vi "Arttu_v09_97.vi"() -> ()   [LabVIEW 2016]
uses:
  x64/Debug/BERTTA.dll
panel:
  out "element":bool
  out "Started:":string
  in  "SHUTDOWN":bool
  in  "MASTER CONTROL":bool
  in  "Tab Control":T1(tab)
  out "Output File":path caption="selected path"
  in  "Browse folder":path=path "" caption="start path"
  in  "Read Seq":bool
  in  "Save Seq":bool
  in  "Configuration file":path=path "C:/Users/shresplab/Desktop/ArttuConfiguration.lvm" caption="Filename"
  in  "OK Button 2":bool
  out "Boolean":bool
  in  "User (initials)":string
  in  "Project name":string
  in  "Description":string
  out "PUMP1":bool
  out "Target amount":dbl
  out "Scale weight":dbl
  out "Amount now":dbl
  out "Flow rate":dbl
  out "Time to target":dbl format="%<%H:%M:%S>t"
  out "Current step":dbl
  out "Target":dbl
  out "Amount now":dbl
  out "Amount now":dbl
  out "Target":dbl
  out "Current step":dbl
  out "Time to target":dbl format="%<%H:%M:%S>t"
  out "Flow rate":dbl
  out "Amount now":dbl
  out "Scale weight":dbl
  out "Target amount":dbl
  out "PUMP2":bool
  out "Sensor OK 6":bool
  out "Sensor OK 5":bool
  out "Sensor OK 4":bool
  out "Sensor OK 3":bool
  in  "OK Button":bool
  in  "Add comment":string
  out "PUMP3":bool
  out "Target amount":dbl
  out "Scale weight":dbl
  out "Amount now":dbl
  out "Flow rate":dbl
  out "Time to target":dbl format="%<%H:%M:%S>t"
  out "Current step":dbl
  out "Target":dbl
  out "Amount now":dbl
  out "Tr":dbl
  out "Tj in":dbl
  out "Tj out":dbl
  out "T set":dbl
  out "Current step":i32
  out "RPM":dbl
  out "Torque 2":dbl
  out "Waveform Chart 5":dynamicdata(graph)
  out "Waveform Chart 6":dynamicdata(graph)
  out "Waveform Chart 7":dynamicdata(graph)
  in  "Tab Control 2":T2(tab)
  out "Waveform Chart 3":dynamicdata(graph)
  out "Waveform Chart 8":dynamicdata(graph)
  out "Waveform Chart 11":dynamicdata(graph)
  out "Waveform Chart 13":dynamicdata(graph)
  out "Waveform Chart 9":dynamicdata(graph)
  out "Table":string[][](table)=[["14.8.2017 18.06.59", "0,000000", "417,670000", "-0,150000", "1,000000", "22,220000", "23,366837", "23,574959", "23,985852", "23,690000", "240,000000", "4,000000", "0,000000", "397,000000", "-397,000000", "1,000000"], ["14.8.2017 18.07.06", "0,000000", "417,640000", "-0,120000", "1,000000", "22,220000", "23,763115", "23,906257", "23,985694", "23,680000", "240,000000", "4,000000", "0,000000", "397,000000", "-397,000000", "1,000000"], ["14.8.2017 18.07.13", "0,000000", "417,640000", "-0,120000", "1,000000", "22,220000", "23,965922", "24,013440", "23,984906", "23,670000", "240,000000", "4,100000", "3,000000", "397,000000", "-397,000000", "1,000000"], ["14.8.2017 18.07.21", "0,000000", "417,640000", "-0,120000", "1,000000", "22,220000", "23,943860", "23,900110", "23,987113", "23,670000", "240,000000", "4,000000", "0,000000", "397,000000", "-397,000000", "1,000000"], ["14.8.2017 18.07.28", "0,000000", "417,640000", "-0,120000", "1,000000", "22,220000", "23,736328", "23,600018", "23,989004", "23,660000", "240,000000", "4,000000", "0,000000", "397,000000", "-397,000000", "1,000000"], ["14.8.2017 18.07.36", "0,000000", "417,640000", "-0,120000", "1,000000", "22,220000", "23,480910", "23,324538", "23,991053", "23,660000", "240,000000", "4,000000", "0,000000", "397,000000", "-397,000000", "1,000000"], ["14.8.2017 18.07.43", "0,000000", "417,640000", "-0,120000", "2,000000", "22,220000", "23,195579", "23,008270", "23,999093", "23,650000", "240,000000", "4,000000", "0,000000", "397,000000", "-397,000000", "1,000000"], ["14.8.2017 18.07.51", "0,000000", "417,650000", "-417,650000", "1,000000", "22,220000", "22,862541", "22,649021", "24,003979", "23,650000", "240,000000", "4,000000", "0,000000", "397,000000", "-397,000000", "2,000000"], ["14.8.2017 18.07.58", "0,000000", "417,640000", "0,010000", "1,000000", "22,220000", "22,541353", "22,354878", "24,005398", "23,650000", "240,000000", "4,000000", "0,000000", "397,000000", "-397,000000", "1,000000"], ["14.8.2017 18.08.06", "0,000000", "417,640000", "0,010000", "1,000000", "22,220000", "22,347931", "22,253738", "24,007605", "23,640000", "240,000000", "4,100000", "0,000000", "397,000000", "-397,000000", "1,000000"], ["14.8.2017 18.08.13", "0,000000", "417,640000", "0,010000", "1,000000", "22,220000", "22,329030", "22,302102", "24,006028", "23,640000", "240,000000", "4,000000", "0,000000", "395,820000", "-395,820000", "1,000000"], ["14.8.2017 18.08.20", "0,000000", "417,640000", "0,010000", "1,000000", "22,220000", "22,466849", "22,511320", "24,002403", "23,630000", "240,000000", "4,000000", "0,000000", "395,830000", "-0,010000", "1,000000"], ["14.8.2017 18.08.28", "0,000000", "417,640000", "0,010000", "1,000000", "22,220000", "22,707062", "22,835101", "24,000984", "23,620000", "240,000000", "4,000000", "0,000000", "395,830000", "-0,010000", "1,000000"], ["14.8.2017 18.08.35", "0,000000", "417,640000", "0,010000", "1,000000", "22,220000", "23,054104", "23,232979", "24,001299", "23,600000", "240,000000", "4,000000", "0,000000", "395,830000", "-0,010000", "1,000000"], ["14.8.2017 18.08.43", "0,000000", "417,640000", "0,010000", "1,000000", "22,220000", "23,412371", "23,522793", "24,002560", "23,590000", "240,000000", "4,000000", "0,000000", "395,820000", "0,000000", "1,000000"], ["14.8.2017 18.08.51", "0,000000", "417,640000", "0,010000", "1,000000", "22,220000", "23,596247", "23,656125", "24,003821", "23,580000", "240,000000", "4,000000", "0,000000", "395,820000", "0,000000", "1,000000"]]
  out "Boolean 4":bool
  out "Boolean 3":bool
  out "Boolean 2":bool
  in  "Reset 6":bool
  in  "Manual/Ramp":bool=TRUE
  in  "Array":dbl[][](array[numeric])=[[20.0, 0.0], [20.0, 0.0], [20.0, 0.0]]
  in  "?":bool
  in  "Time":dbl format="Time to target (min):                %#_g"
  out "Current temp":dbl format="Current temperature (S1):   %#_6g"
  in  "OK Button 3":bool
  in  "T ext / T ext 2":enum32{"Sensor 1", "Sensor 2"}(radio)
  out "Sensor OK":bool
  in  "T fail":dbl=20.0 format="Failsafe temperature:              %#_g"
  in  "Setpoint":dbl=20.0 format="Temperature target:                %#_6g"
  in  "Manual select":T3(radio)
  out "Waveform Chart":dynamicdata(graph)
  out "T external 2":dbl format="Current temperature (S2):    %#_g"
  in  "UPDATE TEMP":bool
  out "Led11 5":bool
  out "RPM":dbl format="%_4f"
  out "Led10 3":bool
  out "Led9 3":bool
  out "Led8 3":bool
  out "Led7 3":bool
  out "Led6 3":bool
  out "Led5 3":bool
  out "Led4 3":bool
  out "Led3 3":bool
  out "Led2 3":bool
  out "Led1 3":bool
  in  "PumpSeq 4":dbl[][](array[numeric])=[[0.0, 0.0, 0.0, 0.0, 0.0, 0.0, 0.0, 0.0, 0.0, 0.0], [0.0, 0.0, 0.0, 0.0, 0.0, 0.0, 0.0, 0.0, 0.0, 0.0], [0.0, 0.0, 0.0, 0.0, 0.0, 0.0, 0.0, 0.0, 0.0, 0.0], [0.0, 0.0, 0.0, 0.0, 0.0, 0.0, 0.0, 0.0, 0.0, 0.0], [0.0, 0.0, 0.0, 0.0, 0.0, 0.0, 0.0, 0.0, 0.0, 0.0], [0.0, 0.0, 0.0, 0.0, 0.0, 0.0, 0.0, 0.0, 0.0, 0.0], [0.0, 0.0, 0.0, 0.0, 0.0, 0.0, 0.0, 0.0, 0.0, 0.0], [0.0, 0.0, 0.0, 0.0, 0.0, 0.0, 0.0, 0.0, 0.0, 0.0], [0.0, 0.0, 0.0, 0.0, 0.0, 0.0, 0.0, 0.0, 0.0, 0.0], [0.0, 0.0, 0.0, 0.0, 0.0, 0.0, 0.0, 0.0, 0.0, 0.0]]
  in  "?":bool
  out "Flow rate (g/min)":dbl
  out "Scale reading":dbl
  out "Step amount now":dbl
  in  "Grams / min":dbl
  out "Waveform Chart 14":dynamicdata(graph)
  in  "?":bool
  out "Total amount now":dbl
  out "Led11 4":bool
  in  "Reset 5":bool
  out "Elapsed / step":i32
  out "Time to target":dbl format="%<%H:%M:%S>t"
  in  "OK Button 4":bool
  out "Led11":bool
  out "RPM":dbl format="%_4f"
  out "Led10":bool
  out "Led9":bool
  out "Led8":bool
  out "Led7":bool
  out "Led6":bool
  out "Led5":bool
  out "Led4":bool
  out "Led3":bool
  out "Led2":bool
  out "Led1":bool
  in  "PumpSeq 2":dbl[][](array[numeric])=[[0.0, 0.0, 0.0, 0.0, 0.0, 0.0, 0.0, 0.0, 0.0, 0.0], [0.0, 0.0, 0.0, 0.0, 0.0, 0.0, 0.0, 0.0, 0.0, 0.0], [0.0, 0.0, 0.0, 0.0, 0.0, 0.0, 0.0, 0.0, 0.0, 0.0], [0.0, 0.0, 0.0, 0.0, 0.0, 0.0, 0.0, 0.0, 0.0, 0.0], [0.0, 0.0, 0.0, 0.0, 0.0, 0.0, 0.0, 0.0, 0.0, 0.0], [0.0, 0.0, 0.0, 0.0, 0.0, 0.0, 0.0, 0.0, 0.0, 0.0], [0.0, 0.0, 0.0, 0.0, 0.0, 0.0, 0.0, 0.0, 0.0, 0.0], [0.0, 0.0, 0.0, 0.0, 0.0, 0.0, 0.0, 0.0, 0.0, 0.0], [0.0, 0.0, 0.0, 0.0, 0.0, 0.0, 0.0, 0.0, 0.0, 0.0], [0.0, 0.0, 0.0, 0.0, 0.0, 0.0, 0.0, 0.0, 0.0, 0.0]]
  in  "?":bool
  out "Flow rate (g/min)":dbl
  out "Scale reading":dbl
  out "Step amount now":dbl
  in  "Grams / min":dbl
  out "Waveform Chart 10":dynamicdata(graph)
  in  "?":bool
  out "Total amount now":dbl
  out "Led11":bool
  in  "Reset 3":bool
  out "Elapsed / step":i32
  out "Time to target":dbl format="%<%H:%M:%S>t"
  in  "OK Button 5":bool
  out "Led11 3":bool
  out "RPM":dbl format="%_4f"
  out "Led10 2":bool
  out "Led9 2":bool
  out "Led8 2":bool
  out "Led7 2":bool
  out "Led6 2":bool
  out "Led5 2":bool
  out "Led4 2":bool
  out "Led3 2":bool
  out "Led2 2":bool
  out "Led1 2":bool
  in  "PumpSeq 3":dbl[][](array[numeric])=[[0.0, 0.0, 0.0, 0.0, 0.0, 0.0, 0.0, 0.0, 0.0, 0.0], [0.0, 0.0, 0.0, 0.0, 0.0, 0.0, 0.0, 0.0, 0.0, 0.0], [0.0, 0.0, 0.0, 0.0, 0.0, 0.0, 0.0, 0.0, 0.0, 0.0], [0.0, 0.0, 0.0, 0.0, 0.0, 0.0, 0.0, 0.0, 0.0, 0.0], [0.0, 0.0, 0.0, 0.0, 0.0, 0.0, 0.0, 0.0, 0.0, 0.0], [0.0, 0.0, 0.0, 0.0, 0.0, 0.0, 0.0, 0.0, 0.0, 0.0], [0.0, 0.0, 0.0, 0.0, 0.0, 0.0, 0.0, 0.0, 0.0, 0.0], [0.0, 0.0, 0.0, 0.0, 0.0, 0.0, 0.0, 0.0, 0.0, 0.0], [0.0, 0.0, 0.0, 0.0, 0.0, 0.0, 0.0, 0.0, 0.0, 0.0], [0.0, 0.0, 0.0, 0.0, 0.0, 0.0, 0.0, 0.0, 0.0, 0.0]]
  in  "?":bool
  out "Flow rate (g/min)":dbl
  out "Scale reading":dbl
  out "Step amount now":dbl
  in  "Grams / min":dbl
  out "Waveform Chart 12":dynamicdata(graph)
  in  "?":bool
  out "Total amount now":dbl
  out "Led11 2":bool
  in  "Reset 4":bool
  out "Elapsed / step":i32
  out "Time to target":dbl format="%<%H:%M:%S>t"
  in  "OK Button 6":bool
  in  "?":bool
  in  "Scale port":dbl=3.0
  out "Waveform Chart 15":dynamicdata(graph)
  in  "?":bool
  in  "OK Button 8":bool
  in  "Remote / Manual":bool
  in  "Set RPM":i32
  out "RPM":dbl
  out "Torque":dbl
  out "Waveform Chart 4":dynamicdata(graph)
  in  "OK Button 7":bool
  out "PortDev out":dbl[](array[numeric])
  in  "Save PortDev":bool
  out "PortDev in":dbl[](array[numeric])
  in  "dev1":i32
  in  "dev2":i32
  in  "dev3":i32
  in  "dev4":i32
  in  "dev5":i32
  in  "dev6":i32
  in  "dev8":i32
  in  "port1":i32
  in  "port2":i32
  in  "port3":i32
  in  "port4":i32
  in  "port5":i32
  in  "port6":i32
  in  "port7":i32
  in  "port8":i32
  in  "dev7":i32
  in  "Treshold (T/C)":dbl=0.5
  out "DAQ 9217 (PT100)":errorcluster
  out "Config File":dbl[][](array[numeric])
  in  "Temp Control":tag="cDAQ9188XT-1C3BEFEMod1"
  in  "PAM Control":tag="cDAQ9188XT-1C3BEFEMod7"
  # "Temperature sensor:"
  # "Manual control:"
  # "PUMP & SCALE 1"
  # "STEP"
  # "TOTAL"
  # "PUMP & SCALE 2"
  # "STEP"
  # "TOTAL"
  # "PUMP & SCALE 3"
  # "STEP"
  # "TOTAL"
  # "Temperature control parameter"
  # "Secondary temperature sensor"
  # "Temp target"
  # "Time target"
  # "Grams    /   min"
  # "End of sequence"
  # "Manual control"
  # "Grams    /   min"
  # "End of sequence"
  # "Manual control"
  # "Grams    /   min"
  # "End of sequence"
  # "Manual control"
  # "PAM control"
  # "dev1 and dev2 always to port1 and 2\nport1 = port2 = Lauda\n\ndev3 and dev4 always to port3 and port4\nport3 = port4 = Heidolph"
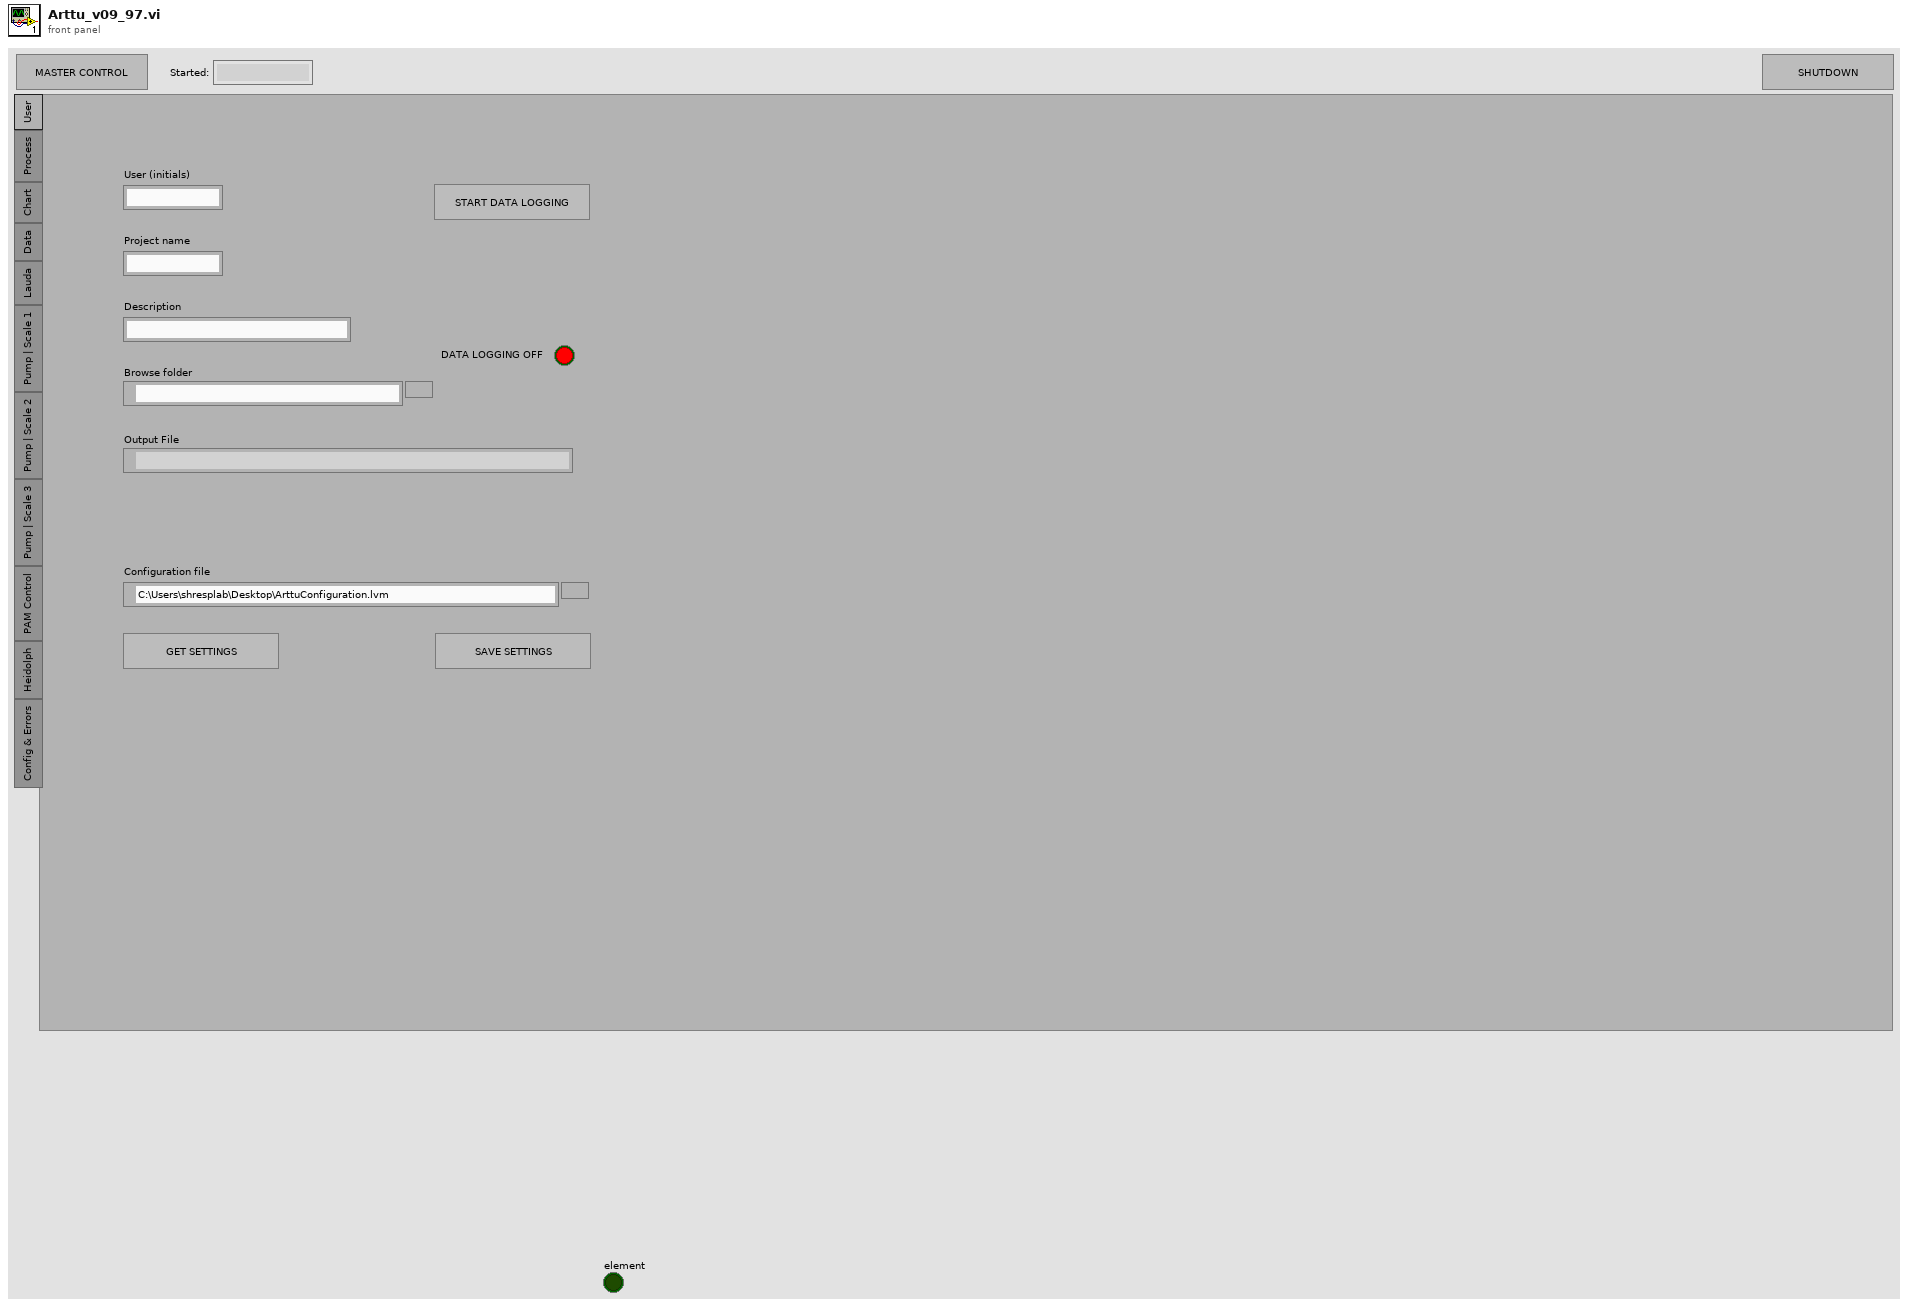
[diagram p1: front panel]
types:
  T1 = enum32{"User", "Process", "Chart", "Data", "Lauda", "Pump | Scale 1", "Pump | Scale 2", "Pump | Scale 3", "PAM Control", "Heidolph", "Config & Errors"}
  T2 = enum32{"Temperatures", "Scale / Pump 1", "Scale / Pump 2", "Scale / Pump 3", "RPM / torque"}
  T3 = enum32{"Reactor temperature", "Jacket temperature"}
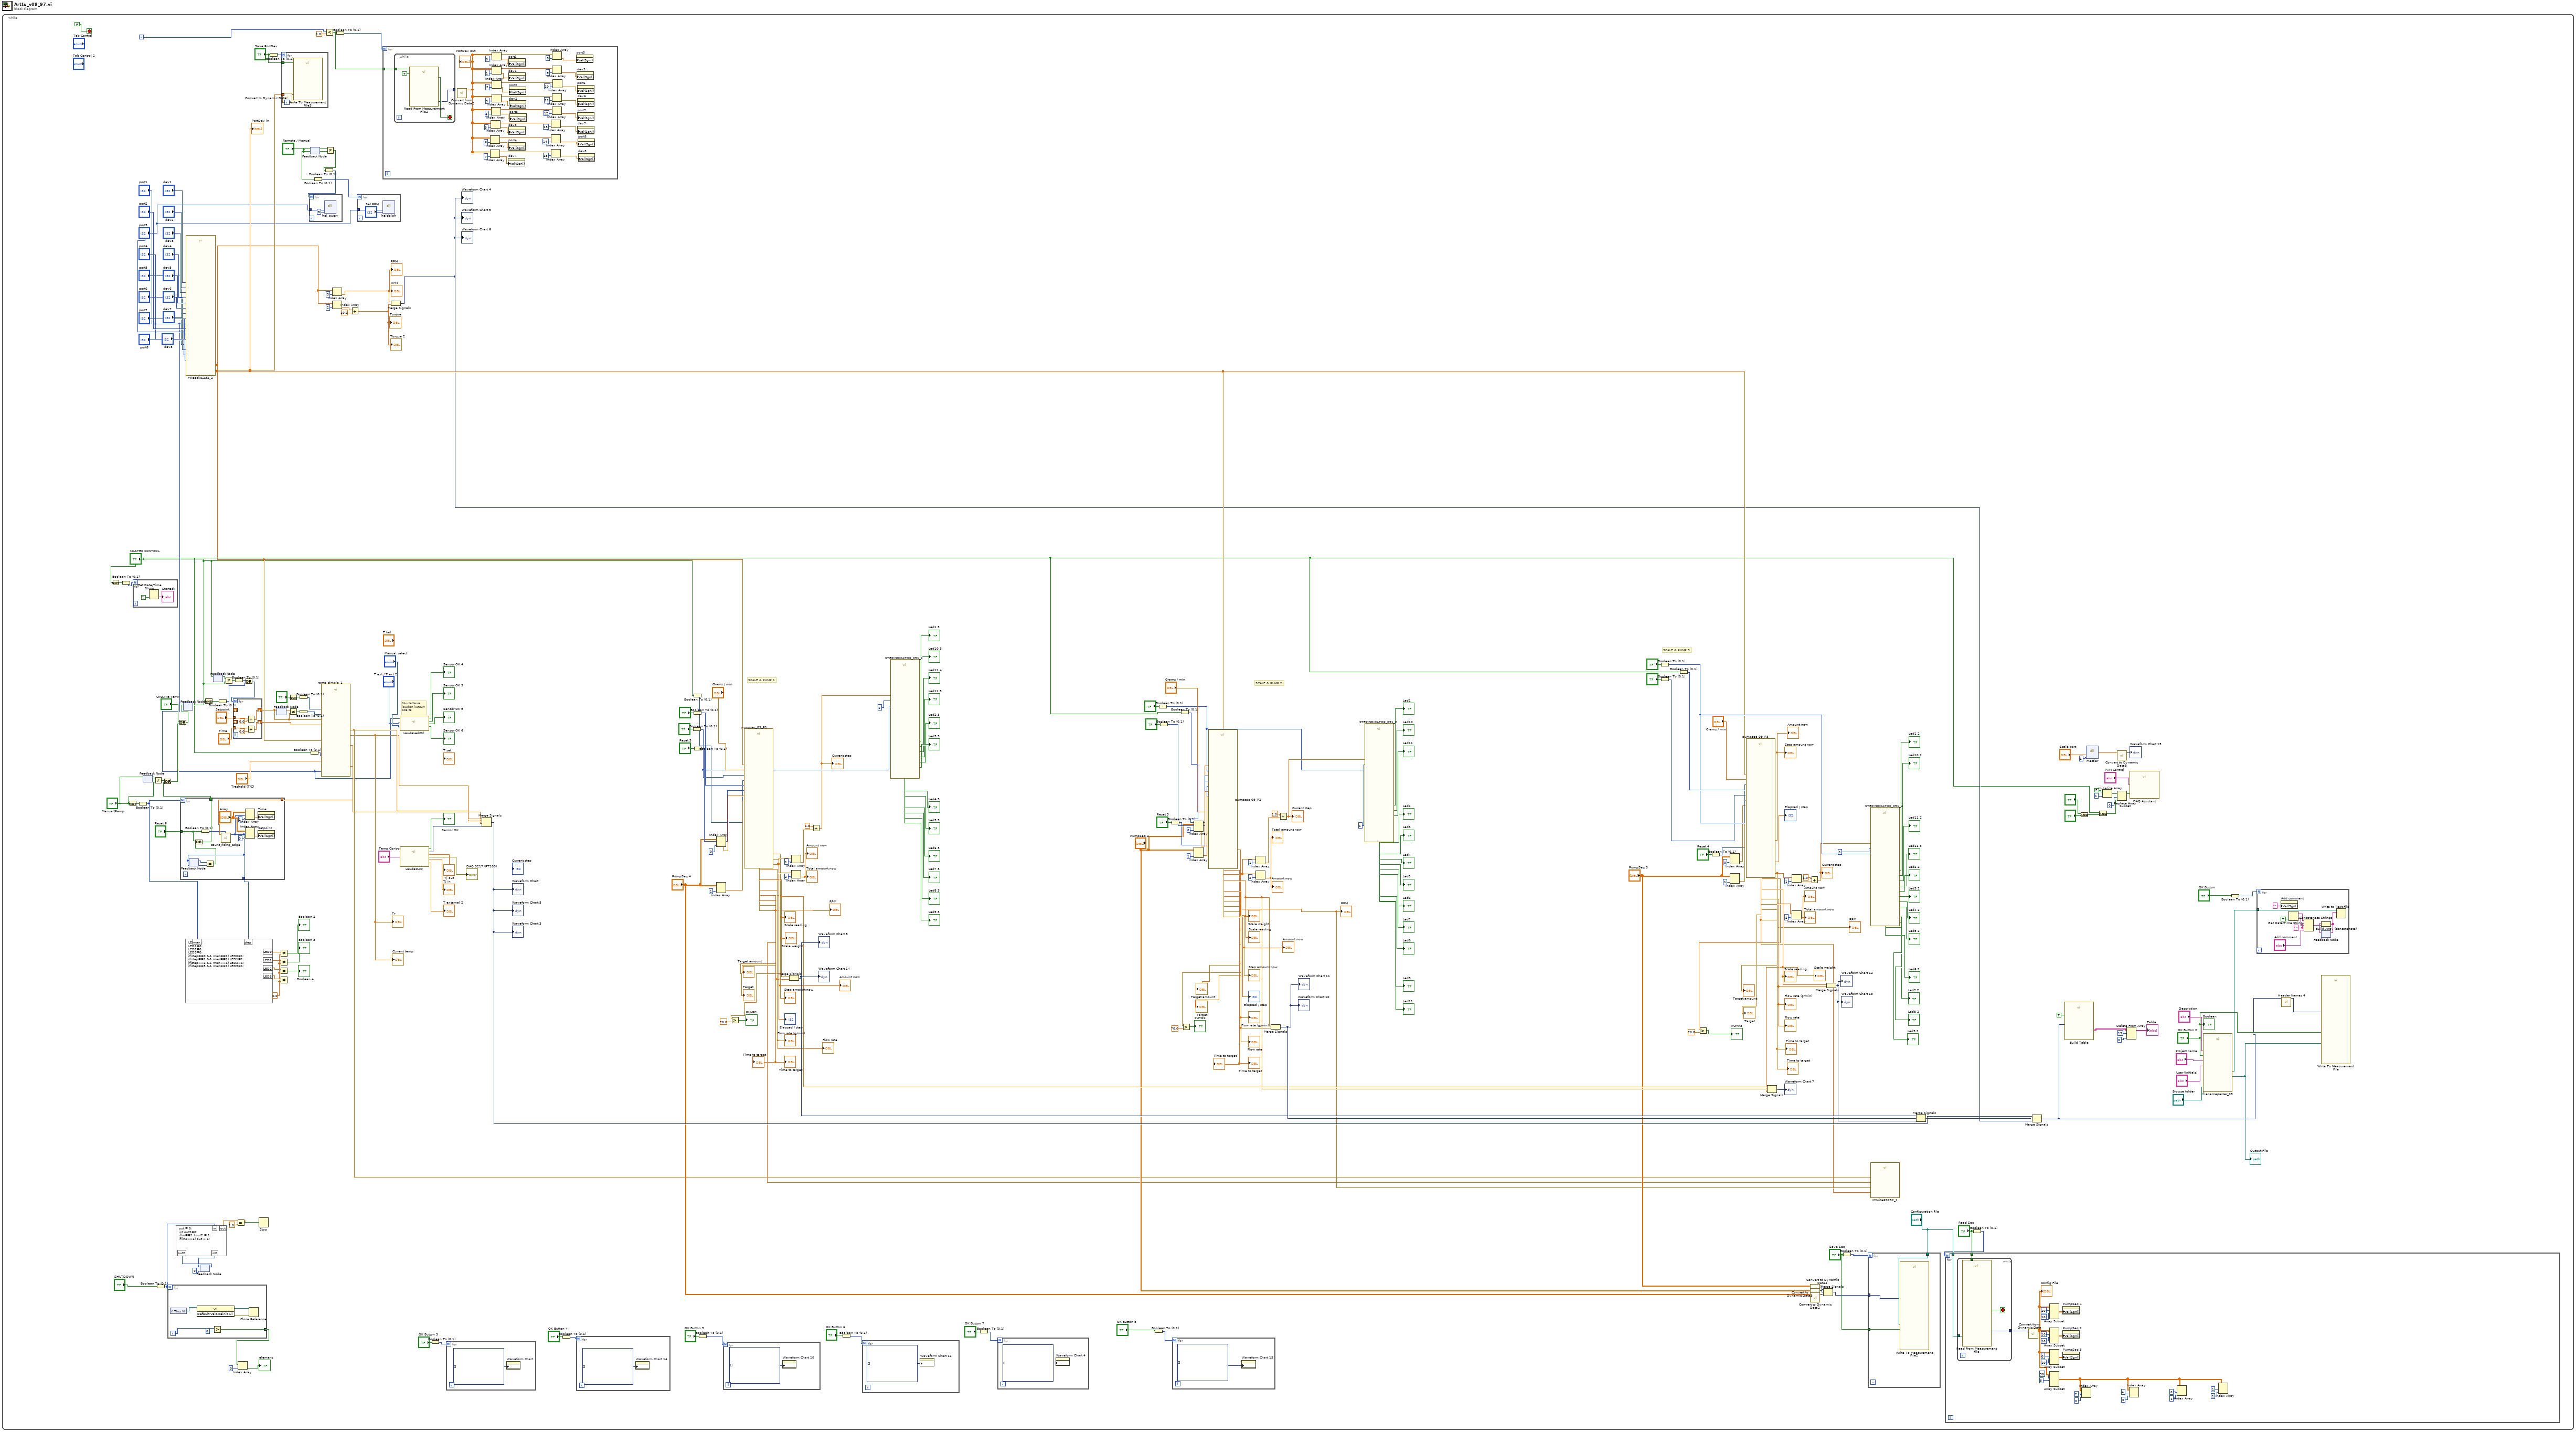
[diagram p0: block diagram]
diagram:
  n1 = while {
    i -> [w61]
    stop <- FALSE stop-if-true
    w47 = 0.0 ("y")
    # "Muutettava\nlaudan kutsun \nosalta"
    # "SCALE & PUMP 1"
    # "SCALE & PUMP 3"
    # "SCALE & PUMP 2"
    n2 = Not(x="MASTER CONTROL") -> (.not. x?=w290:bool)
    n3 = Boolean To (0,1)(Boolean=w290) -> (0, 1=w291:i16)
    n4 = Not(x="Manual/Ramp") -> (.not. x?=w54:bool)
    n5 = for {
      N: w291 -> [_]
      n6 = Get Date/Time String(want seconds? (F)=TRUE) -> (time string=→"Started:":string)  [unwired: 2 in, 1 out]
    }
    n7 = Boolean To (0,1)(Boolean=w54) -> (0, 1=w36:i16)
    n8 = feedback #1() -> (w42:bool)  [unwired: 1 in]
    n9 = feedback-in #1("Manual/Ramp") -> ()
    n10 = Not Equal?(x=w42, y="Manual/Ramp") -> (x != y?=w39:bool)
    n11 = Boolean To (0,1)(Boolean="SHUTDOWN") -> (0, 1=w275:i16)
    n12 = for {
      N: w275 -> [_]
      tunnel: [w407] -> w289 mode=indexing
      i -> [w409]
      n13 = control-ref of="This VI"() -> (w412:refnum<vi>)
      n14 = invoke class="VI" method="Default Vals.Reinit All"(reference=w412) -> (reference out=w410:refnum<vi>, error out=w411:errorcluster)  [unwired: 2 in, 1 out]
      n15 = Greater?(x=w409, y=0) -> (0:w407:bool)
      n16 = Close Reference(reference=w410, error in (no error)=w411) -> ()  [unwired: 1 out]
    }
    n17 = feedback #2() -> (w34:bool)  [unwired: 1 in]
    n18 = call "MReadRS232_2.vi"("port1"="port1", "dev1"="dev1", "port2"="port2", "dev2"="dev2", "port3"="port3", "dev7"="dev7", "dev8"="dev8", "port7"="port7", "port8"="port8", "dev5"="dev5", "port5"="port5", "dev4"="dev4", "dev6"="dev6", "port6"="port6", "port4"="port4", "dev3"="dev3") -> ("output array"=w65:dbl[], "params"=w26:dbl[])  [unwired: 2 in]
    "PortDev in" <- w65
    n19 = feedback #3(0) -> (w273:i32)
    n20 = formula code="out = 0;\nint out2=0;\nif(in==1 ) out2 = 1;\nif(in2==1) out = 1;"("in"=w275, "in2"=w273) -> ("out"=w277:dbl, "out2"=w274:i32)
    n21 = feedback-in #3(w274) -> ()
    n22 = And(x="MASTER CONTROL", y=w34) -> (x .and. y?=w92:bool)
    n23 = feedback #4() -> (w83:bool)  [unwired: 1 in]
    n24 = feedback-in #4("MASTER CONTROL") -> ()
    n25 = Boolean To (0,1)(Boolean=w92) -> (0, 1=w81:i16)
    n26 = Not Equal?(x=w83, y="MASTER CONTROL") -> (x != y?=w82:bool)
    n27 = Boolean To (0,1)(Boolean=w82) -> (0, 1=w80:i16)
    n28 = Equal?(x=w277, y=1.0) -> (x = y?=w276:bool)
    n29 = Index Array(array=w289, index=0) -> (element=→"element":bool)
    n30 = Or(x=w80, y=w81) -> (x .or. y?=w79:i16)
    n31 = for {
      N: w79 -> [_]
      tunnel: "Time" -> [w359]
      shift-right: [w358] -> w93
      shift-left: _ -> [_]
      tunnel: "Setpoint" -> [w356]
      shift-right: [w355] -> w90
      shift-left: _ -> [_]
      n32 = Add(x=w356, y=0.0) -> (x+y=w355:dbl)
      n33 = Add(x=w359, y=0.0) -> (x+y=w358:dbl)
    }
    n34 = Stop(stop? (T)=w276) -> ()
    n35 = Boolean To (0,1)(Boolean="Save PortDev") -> (0, 1=w64:i16)
    n36 = feedback-in #5(w90) -> ()
    n37 = feedback #5() -> (w91:dbl)  [unwired: 1 in]
    n38 = for {
      N: w64 -> [_]
      tunnel: w65 -> [w354]
      tunnel: "Save PortDev" -> [w352]
      n39 = call "Convert to Dynamic Data"("Array"=w354) -> ("Dynamic Data Type"=w353:dynamicdata)  [unwired: 3 in]
      n40 = call "Write To Measurement File3"("Signals"=w353, "Reset"=w352) -> ()  [unwired: 15 in, 3 out]
    }
    n41 = Not(x="?") -> (.not. x?=w86:bool)
    n42 = Not Equal?(x=w91, y=w90) -> (x != y?=w89:bool)
    n43 = Boolean To (0,1)(Boolean=w86) -> (0, 1=w88:i16)
    n44 = Boolean To (0,1)(Boolean=w89) -> (0, 1=w84:i16)
    n45 = Boolean To (0,1)(Boolean="MASTER CONTROL") -> (0, 1=w85:i16)
    n46 = feedback-in #6("Remote / Manual") -> ()
    n47 = feedback #6() -> (w31:bool)  [unwired: 1 in]
    n48 = Boolean To (0,1)(Boolean="Remote / Manual") -> (0, 1=w29:i16)
    n49 = call "ramp_simple_1.vi"("pause"=w88, "time_set"=w93, "array"=w26, "reset"=w84, "master"=w85, "T_sp"=w90, "treshold"="Treshold (T/C)", "port"="port1") -> ("Tin"=w96:dbl, "Tr"=w97:dbl, "target_reached"=w52:dbl, "T control"=w98:dbl)  [unwired: 3 in, 1 out]
    "Tr" <- w97
    "Current temp" <- w97
    n50 = for {
      N: w36 -> [_]
      tunnel: w52 -> [w311]
      tunnel: [w301] -> w40
      tunnel: "Reset 6" -> [w303]
      tunnel: [w304] -> w43
      n51 = feedback #7() -> (w305:i32)  [unwired: 1 in]
      n52 = Boolean To (0,1)(Boolean=w303) -> (0, 1=w306:i16)
      n53 = call "count_rising_edge.vi"("reset"=w306, "target_reached"=w311) -> ("element 2"=w304:i32)  [unwired: 9 in]
      n54 = feedback-in #7(w304) -> ()
      n55 = Not Equal?(x=w305, y=w304) -> (x != y?=w302:bool)
      n56 = Or(x=w303, y=w302) -> (x .or. y?=w301:bool)
      n57 = Index Array(array="Array", index (row)=w304, index (col)=1 ("disabled index (col)")) -> (element=w307:dbl)
      n58 = Index Array(array="Array", index (row)=w304, index (col)=0 ("disabled index (col)")) -> (element=w308:dbl)
      n59 = property on="Time" class="DigNum (strict)"("Val(Sgnl)"=w307) -> ()  [unwired: 2 in, 2 out]
      n60 = property on="Setpoint" class="DigNum (strict)"("Val(Sgnl)"=w308) -> ()  [unwired: 2 in, 2 out]
    }
    n61 = Or(x=w39, y=w40) -> (x .or. y?=w38:bool)
    n62 = Or(x="UPDATE TEMP", y=w38) -> (x .or. y?=w35:bool)
    n63 = feedback-in #2(w35) -> ()
    n64 = formula code="LED0=0;\nLED1=0;\nLED2=0;\nLED3=0;\nif(step==0 && man==1) LED0=1;\nif(step==1 && man==1) LED1=1;\nif(step==2 && man==1) LED2=1;\nif(step==3 && man==1) LED3=1;"("step"=w43, "man"=w36) -> ("LED0"=w51:dbl, "LED1"=w50:dbl, "LED2"=w49:dbl, "LED3"=w48:dbl)
    n65 = Not Equal?(x=w51, y=w47) -> (x != y?=→"Boolean 2":bool)
    n66 = Not Equal?(x=w50, y=w47) -> (x != y?=→"Boolean 3":bool)
    n67 = Not Equal?(x=w49, y=w47) -> (x != y?=→"Boolean 4":bool)
    n68 = Not Equal?(x=w48, y=w47) -> ()  [unwired: 1 out]
    n69 = Less?(x=w61, y=1.0) -> (x < y?=w59:bool)
    n70 = Not Equal?(x=w31, y="Remote / Manual") -> (x != y?=w30:bool)
    n71 = Boolean To (0,1)(Boolean=w30) -> (0, 1=w32:i16)
    n72 = for {
      N: w32 -> [_]
      tunnel: "port3" -> [w299]
      n73 = dll-call lib="C:/Users/shresplab/OneDrive - Kemira Oyj/Documents/GitHub/Bertta/BERTTA/x64/Debug/BERTTA.dll" fn="hei_query"("port"=w299, "q"=5) -> ()  [unwired: 6 in, 2 out]
    }
    n74 = Index Array(array=w26, index=3) -> (element=w23:dbl)
    "RPM" <- w23
    "RPM" <- w23
    n75 = Index Array(array=w26, index=2) -> (element=w25:dbl)
    n76 = Boolean To (0,1)(Boolean=w59) -> (0, 1=w60:i16)
    n77 = Divide(x=w25, y=10.0) -> (x/y=w22:dbl)
    "Torque" <- w22
    "Torque 2" <- w22
    n78 = for {
      N: w29 -> [_]
      tunnel: "port3" -> [w297]
      n79 = dll-call lib="C:/Users/shresplab/OneDrive - Kemira Oyj/Documents/GitHub/Bertta/BERTTA/x64/Debug/BERTTA.dll" fn="heidolph"("port"=w297, "speed"="Set RPM") -> ()  [unwired: 6 in, 2 out]
    }
    n80 = for {
      N: w60 -> [_]
      tunnel: w59 -> [w347]
      n81 = while {
        tunnel: [w350] -> w346
        tunnel: w347 -> [w348]
        stop <- w351 stop-if-true
        n82 = call "Read From Measurement File2"("Enable"=TRUE, "Reset"=w348) -> ("Signals"=w350:dynamicdata, "EOF?"=w351:bool)  [unwired: 4 in, 4 out]
      }
      n83 = call "Convert from Dynamic Data2"("Dynamic Data Type"=w346) -> ("Array"=w329:dbl[])  [unwired: 3 in]
      "PortDev out" <- w329
      n84 = Index Array(array=w329, index=6) -> (element=w322:dbl)
      n85 = Index Array(array=w329, index=7) -> (element=w321:dbl)
      n86 = Index Array(array=w329, index=5) -> (element=w323:dbl)
      n87 = Index Array(array=w329, index=4) -> (element=w324:dbl)
      n88 = Index Array(array=w329, index=0) -> (element=w328:dbl)
      n89 = Index Array(array=w329, index=1) -> (element=w327:dbl)
      n90 = Index Array(array=w329, index=3) -> (element=w325:dbl)
      n91 = Index Array(array=w329, index=2) -> (element=w326:dbl)
      n92 = property on="dev4" class="DigNum (strict)"("Val(Sgnl)"=w321) -> ()  [unwired: 2 in, 2 out]
      n93 = property on="dev3" class="DigNum (strict)"("Val(Sgnl)"=w323) -> ()  [unwired: 2 in, 2 out]
      n94 = property on="port4" class="DigNum (strict)"("Val(Sgnl)"=w322) -> ()  [unwired: 2 in, 2 out]
      n95 = property on="port1" class="DigNum (strict)"("Val(Sgnl)"=w328) -> ()  [unwired: 2 in, 2 out]
      n96 = property on="dev1" class="DigNum (strict)"("Val(Sgnl)"=w327) -> ()  [unwired: 2 in, 2 out]
      n97 = property on="port2" class="DigNum (strict)"("Val(Sgnl)"=w326) -> ()  [unwired: 2 in, 2 out]
      n98 = property on="dev2" class="DigNum (strict)"("Val(Sgnl)"=w325) -> ()  [unwired: 2 in, 2 out]
      n99 = property on="port3" class="DigNum (strict)"("Val(Sgnl)"=w324) -> ()  [unwired: 2 in, 2 out]
      n100 = Index Array(array=w329, index=14) -> (element=w314:dbl)
      n101 = Index Array(array=w329, index=15) -> (element=w313:dbl)
      n102 = Index Array(array=w329, index=13) -> (element=w315:dbl)
      n103 = Index Array(array=w329, index=12) -> (element=w316:dbl)
      n104 = Index Array(array=w329, index=8) -> (element=w320:dbl)
      n105 = Index Array(array=w329, index=9) -> (element=w319:dbl)
      n106 = Index Array(array=w329, index=11) -> (element=w317:dbl)
      n107 = Index Array(array=w329, index=10) -> (element=w318:dbl)
      n108 = property on="port5" class="DigNum (strict)"("Val(Sgnl)"=w320) -> ()  [unwired: 2 in, 2 out]
      n109 = property on="dev5" class="DigNum (strict)"("Val(Sgnl)"=w319) -> ()  [unwired: 2 in, 2 out]
      n110 = property on="port6" class="DigNum (strict)"("Val(Sgnl)"=w318) -> ()  [unwired: 2 in, 2 out]
      n111 = property on="dev6" class="DigNum (strict)"("Val(Sgnl)"=w317) -> ()  [unwired: 2 in, 2 out]
      n112 = property on="port7" class="DigNum (strict)"("Val(Sgnl)"=w316) -> ()  [unwired: 2 in, 2 out]
      n113 = property on="dev7" class="DigNum (strict)"("Val(Sgnl)"=w315) -> ()  [unwired: 2 in, 2 out]
      n114 = property on="port8" class="DigNum (strict)"("Val(Sgnl)"=w314) -> ()  [unwired: 2 in, 2 out]
      n115 = property on="dev8" class="DigNum (strict)"("Val(Sgnl)"=w313) -> ()  [unwired: 2 in, 2 out]
    }
    n116 = Merge Signals(w23, w22) -> (w21:dynamicdata)
    "Waveform Chart 4" <- w21
    "Waveform Chart 6" <- w21
    "Waveform Chart 9" <- w21
    n117 = call "LaudaLedCtrl.vi"("Manual select"="Manual select", "T ext / T ext in"="T ext / T ext 2", "Lauda port"="port1") -> ("Sensor OK 5"=→"Sensor OK 5":bool, "Sensor OK 3"=→"Sensor OK 3":bool, "Sensor OK 4"=→"Sensor OK 4":bool, "Sensor OK 6"=→"Sensor OK 6":bool)  [unwired: 5 in]
    n118 = call "LaudaDAQ.vi"("device name"="Temp Control") -> ("error out"=→"DAQ 9217 (PT100)":errorcluster, 1:"Tj out"=→"Tj out":dbl, "data"=w165:dynamicdata, "Sensor OK"=→"Sensor OK":bool, 4:"Tj out"=→"Tj in":dbl, "T external 2"=→"T external 2":dbl)  [unwired: 5 in]
    n119 = Boolean To (0,1)(Boolean="OK Button 3") -> (0, 1=w109:i16)
    n120 = for {
      N: w109 -> [_]
      n121 = property on="Waveform Chart" class="WFChart (strict)"("History Data"=dynamicdata[] []) -> ()  [unwired: 2 in, 2 out]
    }
    n122 = Merge Signals(w98, w97, w96, w165) -> (w166:dynamicdata)
    "Waveform Chart 3" <- w166
    "Waveform Chart" <- w166
    "Waveform Chart 5" <- w166
    n123 = Boolean To (0,1)(Boolean="OK Button 4") -> (0, 1=w107:i16)
    n124 = for {
      N: w107 -> [_]
      n125 = property on="Waveform Chart 14" class="WFChart (strict)"("History Data"=dynamicdata[] []) -> ()  [unwired: 2 in, 2 out]
    }
    n126 = Boolean To (0,1)(Boolean="?") -> (0, 1=w174:i16)
    n127 = Boolean To (0,1)(Boolean="?") -> (0, 1=w178:i16)
    n128 = Boolean To (0,1)(Boolean="MASTER CONTROL") -> (0, 1=w170:i16)
    n129 = Boolean To (0,1)(Boolean="Reset 5") -> (0, 1=w177:i16)
    n130 = Boolean To (0,1)(Boolean="OK Button 5") -> (0, 1=w105:i16)
    n131 = Index Array(array="PumpSeq 4", index (col)=0) -> (element=w182:dbl[])  [unwired: 1 in]
    n132 = Index Array(array="PumpSeq 4", index (col)=1) -> (element=w203:dbl[])  [unwired: 1 in]
    n133 = for {
      N: w105 -> [_]
      n134 = property on="Waveform Chart 10" class="WFChart (strict)"("History Data"=dynamicdata[] []) -> ()  [unwired: 2 in, 2 out]
    }
    n135 = call "pumpsec_09_P1.vi"("reset"=w177, "master"=w170, "manual"=w174, "pause"=w178, "Array"=w26, "Target"=w182, "fr_manual"="Grams / min", "Time"=w203) -> ("pumpCtrl"=w149:dbl, "totaltarget"=→"Target":dbl, "target_step"=→"Target amount":dbl, "REGLO D"=w115:dbl, "time_to_target"=→"Time to target" →"Time to target":dbl, "step_fr"=w126:dbl, "amount_step"=→"Amount now" →"Step amount now":dbl, "Scale"=w161:dbl, "elapsed_step"=→"Elapsed / step":dbl, "params"=w200:dbl[])  [unwired: 8 in, 2 out]
    "Flow rate" <- w126
    "Scale weight" <- w161
    "Scale reading" <- w161
    "Flow rate (g/min)" <- w126
    "RPM" <- w115
    n136 = Greater?(x=w149, y=70.0) -> (0:→"PUMP1":bool)
    n137 = Merge Signals(w161, w126) -> (w169:dynamicdata)
    "Waveform Chart 8" <- w169
    "Waveform Chart 14" <- w169
    n138 = Index Array(array=w200, index=1) -> (element=w197:dbl)
    n139 = Index Array(array=w200, index=2) -> (element=→"Amount now" →"Total amount now":dbl)
    n140 = Add(x=1.0, y=w197) -> (x+y=w127:dbl)
    "Current step" <- w127
    n141 = Boolean To (0,1)(Boolean="OK Button 6") -> (0, 1=w103:i16)
    n142 = for {
      N: w103 -> [_]
      n143 = property on="Waveform Chart 12" class="WFChart (strict)"("History Data"=dynamicdata[] []) -> ()  [unwired: 2 in, 2 out]
    }
    n144 = call "STEPINDICATOR_091_2.vi"("current step"=w127, "enable"=i16 1, "manual"=w174) -> ("Led 8"=→"Led8 3":bool, "Led 10"=→"Led10 3":bool, "Led 11"=→"Led11 4":bool, "Led 7"=→"Led7 3":bool, "Led 1"=→"Led1 3":bool, "Led 6"=→"Led6 3":bool, "Led 2"=→"Led2 3":bool, "Led 12"=→"Led11 5":bool, "Led 5"=→"Led5 3":bool, "Led 4"=→"Led4 3":bool, "Led 3"=→"Led3 3":bool, "Led 9"=→"Led9 3":bool)  [unwired: 1 in]
    n145 = Boolean To (0,1)(Boolean="OK Button 7") -> (0, 1=w101:i16)
    n146 = for {
      N: w101 -> [_]
      n147 = property on="Waveform Chart 4" class="WFChart (strict)"("History Data"=dynamicdata[] []) -> ()  [unwired: 2 in, 2 out]
    }
    n148 = Boolean To (0,1)(Boolean="OK Button 8") -> (0, 1=w17:i16)
    n149 = Boolean To (0,1)(Boolean="?") -> (0, 1=w237:i16)
    n150 = Boolean To (0,1)(Boolean="?") -> (0, 1=w264:i16)
    n151 = Boolean To (0,1)(Boolean="Reset 3") -> (0, 1=w262:i16)
    n152 = for {
      N: w17 -> [_]
      n153 = property on="Waveform Chart 15" class="WFChart (strict)"("History Data"=dynamicdata[] []) -> ()  [unwired: 2 in, 2 out]
    }
    n154 = Boolean To (0,1)(Boolean="MASTER CONTROL") -> (0, 1=w256:i16)
    n155 = Index Array(array="PumpSeq 2", index (col)=0 ("disabled index (col)")) -> (element=w267:dbl[])  [unwired: 1 in]
    n156 = Index Array(array="PumpSeq 2", index (col)=1 ("disabled index (col)")) -> (element=w266:dbl[])  [unwired: 1 in]
    n157 = call "pumpsec_09_P2.vi"("reset"=w262, "master"=w256, "manual"=w237, "pause"=w264, "Array"=w26, "Target"=w267, "fr_manual"="Grams / min", "Time"=w266) -> ("pumpCtrl"=w145:dbl, "totaltarget"=→"Target":dbl, "target_step"=→"Target amount":dbl, "REGLO D"=w114:dbl, "time_to_target"=→"Time to target" →"Time to target":dbl, "step_fr"=w164:dbl, "amount_step"=→"Amount now" →"Step amount now":dbl, "Scale"=w160:dbl, "elapsed_step"=→"Elapsed / step":dbl, "params"=w257:dbl[])  [unwired: 8 in, 2 out]
    "Scale weight" <- w160
    "Flow rate" <- w164
    "Scale reading" <- w160
    "Flow rate (g/min)" <- w164
    "RPM" <- w114
    n158 = Greater?(x=w145, y=70.0) -> (0:→"PUMP2":bool)
    n159 = Index Array(array=w257, index=1) -> (element=w260:dbl)
    n160 = Index Array(array=w257, index=2) -> (element=→"Amount now" →"Total amount now":dbl)
    n161 = Merge Signals(w160, w164) -> (w171:dynamicdata)
    "Waveform Chart 11" <- w171
    "Waveform Chart 10" <- w171
    n162 = Add(x=1.0, y=w260) -> (x+y=w254:dbl)
    "Current step" <- w254
    n163 = call "STEPINDICATOR_091_2.vi"("current step"=w254, "enable"=i16 1, "manual"=w237) -> ("Led 8"=→"Led8":bool, "Led 10"=→"Led10":bool, "Led 11"=→"Led11":bool, "Led 7"=→"Led7":bool, "Led 1"=→"Led1":bool, "Led 6"=→"Led6":bool, "Led 2"=→"Led2":bool, "Led 12"=→"Led11":bool, "Led 5"=→"Led5":bool, "Led 4"=→"Led4":bool, "Led 3"=→"Led3":bool, "Led 9"=→"Led9":bool)  [unwired: 1 in]
    n164 = Boolean To (0,1)(Boolean="?") -> (0, 1=w231:i16)
    n165 = Boolean To (0,1)(Boolean="?") -> (0, 1=w230:i16)
    n166 = Boolean To (0,1)(Boolean="MASTER CONTROL") -> (0, 1=w232:i16)
    n167 = Boolean To (0,1)(Boolean="Reset 4") -> (0, 1=w212:i16)
    n168 = Index Array(array="PumpSeq 3", index (col)=0 ("disabled index (col)")) -> (element=w215:dbl[])  [unwired: 1 in]
    n169 = Index Array(array="PumpSeq 3", index (col)=1 ("disabled index (col)")) -> (element=w214:dbl[])  [unwired: 1 in]
    n170 = call "pumpsec_09_P3.vi"("reset"=w212, "master"=w232, "manual"=w231, "pause"=w230, "Array"=w26, "Target"=w215, "fr_manual"="Grams / min", "Time"=w214) -> ("pumpCtrl"=w142:dbl, "totaltarget"=→"Target":dbl, "target_step"=→"Target amount":dbl, "REGLO D"=w113:dbl, "time_to_target"=→"Time to target" →"Time to target":dbl, "step_fr"=w163:dbl, "amount_step"=→"Amount now" →"Step amount now":dbl, "Scale"=w159:dbl, "elapsed_step"=→"Elapsed / step":dbl, "params"=w205:dbl[])  [unwired: 8 in, 2 out]
    "Scale weight" <- w159
    "Flow rate" <- w163
    "Scale reading" <- w159
    "Flow rate (g/min)" <- w163
    "RPM" <- w113
    n171 = Greater?(x=w142, y=70.0) -> (0:→"PUMP3":bool)
    n172 = Merge Signals(w161, w160, w159) -> (→"Waveform Chart 7":dynamicdata)
    n173 = Index Array(array=w205, index=1) -> (element=w206:dbl)
    n174 = Index Array(array=w205, index=2) -> (element=→"Amount now" →"Total amount now":dbl)
    n175 = Add(x=1.0, y=w206) -> (x+y=w204:dbl)
    "Current step" <- w204
    n176 = call "Convert to Dynamic Data4"("2D Array"="PumpSeq 3") -> ("Dynamic Data Type"=w118:dynamicdata)  [unwired: 3 in]
    n177 = call "Convert to Dynamic Data3"("2D Array"="PumpSeq 2") -> ("Dynamic Data Type"=w120:dynamicdata)  [unwired: 3 in]
    n178 = call "Convert to Dynamic Data2"("2D Array"="PumpSeq 4") -> ("Dynamic Data Type"=w123:dynamicdata)  [unwired: 3 in]
    n179 = Merge Signals(w118, w120, w123) -> (w122:dynamicdata)
    n180 = Merge Signals(w159, w163) -> (w168:dynamicdata)
    "Waveform Chart 13" <- w168
    "Waveform Chart 12" <- w168
    n181 = Boolean To (0,1)(Boolean="Save Seq") -> (0, 1=w117:i16)
    n182 = for {
      N: w117 -> [_]
      tunnel: w122 -> [w405]
      tunnel: "Configuration file" -> [w406]
      tunnel: "Save Seq" -> [w404]
      n183 = call "Write To Measurement File2"("Signals"=w405, "Reset"=w404, "Filename"=w406) -> ()  [unwired: 14 in, 3 out]
    }
    n184 = call "STEPINDICATOR_091_4.vi"("current step"=w204, "enable"=i16 1, "manual"=w231) -> ("Led 8"=→"Led8 2":bool, "Led 10"=→"Led10 2":bool, "Led 11"=→"Led11 2":bool, "Led 7"=→"Led7 2":bool, "Led 1"=→"Led1 2":bool, "Led 6"=→"Led6 2":bool, "Led 2"=→"Led2 2":bool, "Led 12"=→"Led11 3":bool, "Led 5"=→"Led5 2":bool, "Led 4"=→"Led4 2":bool, "Led 3"=→"Led3 2":bool, "Led 9"=→"Led9 2":bool)  [unwired: 1 in]
    n185 = call "MWriteRS232_1.vi"("P3"=w113, "P2"=w114, "P1"=w115, "LAUDA"=w98) -> ()  [unwired: 8 in]
    n186 = Merge Signals(w169, w171, w168) -> (w167:dynamicdata)
    n187 = Boolean To (0,1)(Boolean="Read Seq") -> (0, 1=w116:i16)
    n188 = for {
      N: w116 -> [_]
      tunnel: "Configuration file" -> [w377]
      tunnel: "Read Seq" -> [w376]
      n189 = while {
        tunnel: [w403] -> w399
        tunnel: w377 -> [w402]
        tunnel: w376 -> [w400]
        stop <- w401 stop-if-true
        n190 = call "Read From Measurement File"("Filename"=w402, "Reset"=w400) -> ("Signals"=w403:dynamicdata, "EOF?"=w401:bool)  [unwired: 4 in, 4 out]
      }
      n191 = call "Convert from Dynamic Data"("Dynamic Data Type"=w399) -> ("Array"=w389:dbl[][])  [unwired: 3 in]
      "Config File" <- w389
      n192 = Array Subset(array=w389, index (row)=20 ("index"), length (row)=10 ("length")) -> (w396:dbl[][])  [unwired: 2 in]
      n193 = Array Subset(array=w389, index (row)=10 ("index"), length (row)=10 ("length")) -> (w391:dbl[][])  [unwired: 2 in]
      n194 = Array Subset(array=w389, index (row)=0 ("index"), length (row)=10 ("length")) -> (w390:dbl[][])  [unwired: 2 in]
      n195 = Array Subset(array=w389, index (row)=30 ("index"), length (row)=8 ("length")) -> (w378:dbl[][])  [unwired: 2 in]
      n196 = property on="PumpSeq 4" class="Arr (strict)"("Val(Sgnl)"=w396) -> ()  [unwired: 2 in, 2 out]
      n197 = property on="PumpSeq 2" class="Arr (strict)"("Val(Sgnl)"=w391) -> ()  [unwired: 2 in, 2 out]
      n198 = property on="PumpSeq 3" class="Arr (strict)"("Val(Sgnl)"=w390) -> ()  [unwired: 2 in, 2 out]
      n199 = Index Array(array=w378, index (row)=2, index (col)=0 ("disabled index (col)")) -> ()  [unwired: 1 out]
      n200 = Index Array(array=w378, index (row)=4, index (col)=0 ("disabled index (col)")) -> ()  [unwired: 1 out]
      n201 = Index Array(array=w378, index (row)=0, index (col)=1 ("disabled index (col)")) -> ()  [unwired: 1 out]
      n202 = Index Array(array=w378, index (row)=1, index (col)=1 ("disabled index (col)")) -> ()  [unwired: 1 out]
    }
    n203 = Merge Signals(w166, w167, w21) -> (w57:dynamicdata)
    n204 = call "Build Table"("Include time data"=TRUE, "Signals"=w57) -> ("Table"=w285:string[][])  [unwired: 3 in, 6 out]
    n205 = And(x="?", y="?") -> (x .and. y?=w9:bool)
    n206 = dll-call lib="C:/Users/shresplab/OneDrive - Kemira Oyj/Documents/GitHub/Bertta/BERTTA/x64/Debug/BERTTA.dll" fn="mettler"("port"="Scale port", "msg"=1) -> ("return type"=w2:dbl)  [unwired: 5 in, 2 out]
    n207 = And(x="MASTER CONTROL", y=w9) -> (x .and. y?=w5:bool)
    n208 = Initialize Array(FALSE, 1 ("dimension size")) -> (w7:bool[])
    n209 = Replace Array Subset(array=w7, new element=w5, index=0) -> (w4:bool[])
    n210 = call "Convert to Dynamic Data5"("Double"=w2) -> ("Dynamic Data Type"=→"Waveform Chart 15":dynamicdata)  [unwired: 3 in]
    n211 = Delete From Array(array=w285, length=13, index (col)=0 ("index (row)")) -> (array with subset deleted=→"Table":string[][])  [unwired: 1 in, 1 out]
    n212 = call "DAQ Assistant"("data"=w4, "device name"="PAM Control") -> ()  [unwired: 16 in, 2 out]
    n213 = call "filenameparser_09.vi"("Description"="Description", "start path"="Browse folder", "Project name"="Project name", "User (initials)"="User (initials)", "OK Button in"="OK Button 2") -> ("appended path 2"=w99:path, "appended path"=w281:path)  [unwired: 4 in, 1 out]
    "Output File" <- w99
    n214 = Boolean To (0,1)(Boolean="OK Button") -> (0, 1=w280:i16)
    n215 = for {
      N: w280 -> [_]
      tunnel: w281 -> [w368]
      w372 = " " ("string")
      n216 = property on="Add comment" class="Str"("Val(Sgnl)"="" ("Value (Signaling)")) -> ()  [unwired: 2 in, 2 out]
      n217 = Get Date/Time String(want seconds? (F)=TRUE) -> (date string=w375:string, time string=w373:string)  [unwired: 2 in]
      n218 = Concatenate Strings(w375, w372, w373, w372, "Add comment") -> (w371:string)
      n219 = feedback #8() -> (w370:string[])  [unwired: 1 in]
      n220 = Build Array (concatenate)(w370, w371) -> (w369:string[])
      n221 = feedback-in #8(w369) -> ()
      n222 = Write to Text File(file (use dialog)=w368, text=w369) -> ()  [unwired: 2 in, 3 out]
    }
    n223 = call "Header Names 4.vi"("Dynamic Data"=w57) -> ("Signals Out"=w58:dynamicdata)  [unwired: 10 in]
    n224 = call "Write To Measurement File"("Signals"=w58, "Enable"="OK Button 2", "Filename"=w99) -> ()  [unwired: 14 in, 3 out]
    "Boolean" <- "OK Button 2"
  }
